vi "DVW_Create Array of Refs.vi"(11 "Waveforms":T1[](array[typedef])) -> (3 "Array":T2[](array[typedef]))   [LabVIEW 2015]
uses:
  TypeDefs_Utility/Ref_DVR_Buffer.ctl
  Universal Controls/Waveform_Data.ctl
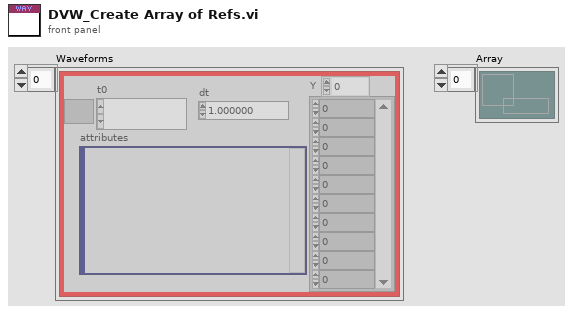
[diagram p1: front panel]
types:
  T1 = typedef "Waveform_Data.ctl" = waveform(dbl)
  T2 = typedef "Ref_DVR_Buffer.ctl" = refnum<data-value>
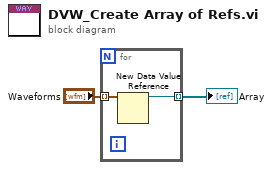
[diagram p0: block diagram]
diagram:
  n1 = for {
    tunnel: "Waveforms" -> [w4] mode=indexing
    tunnel: [w3] -> w2 mode=indexing
    n2 = New Data Value Reference(data value=w4) -> (data value reference=w3:refnum<data-value>)  [unwired: 1 in, 1 out]
  }
  "Array" <- w2
